vi "Error Description.vi"(8 "error in (no error)":errorcluster, 10 "Code":i32) -> (0 "error out":errorcluster, 2 "Description":string)   [LabVIEW 8.6, in "ZTScopeM.lvlib"]
doc: "Query an error code's string description\n\nNote: These are instrument error codes not VISA error codes."
uses:
  ZTScopeM.lvlib
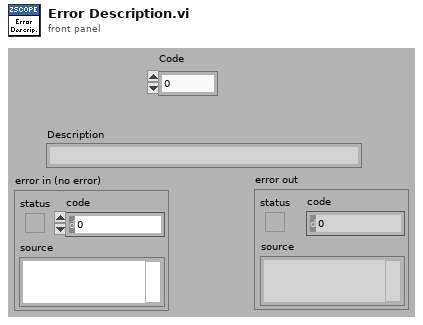
[diagram p1: front panel]
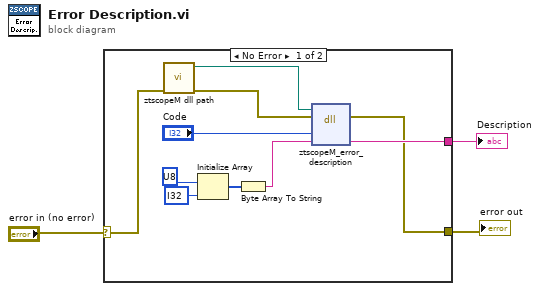
[diagram p0: block diagram]
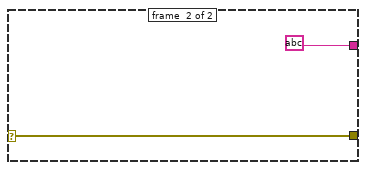
[diagram p2: hidden frame]
diagram:
  n1 = case shown="No Error" "error in (no error)" {
    selector: "error in (no error)" -> [w6 w15]
    tunnel: [w12 string ?] -> w3
    tunnel: [w4 w15] -> w1
    frame #0 {
      n2 = call "ztscopeM dll path.vi"("error in (no error)"=w6) -> ("error out"=w5:errorcluster, "<instrument>.dll path"=w7:path)  [unwired: 9 in]
      n3 = Initialize Array(u8 ?, i32 ? ("dimension size")) -> (w10:u8[])
      n4 = Byte Array To String(unsigned byte array=w10) -> (string=w9:string)
      n5 = dll-call lib="C:/Program Files (x86)/National Instruments/LabVIEW 2013/instr.lib/ztscopem/ztscopeM.dll" fn="ztscopeM_error_description"(path in=w7, error in=w5, "code"="Code", "description"=w9) -> (error out=w4:errorcluster, "description"=w12:string)  [unwired: 3 in, 1 out]
    }
    frame #1 {
    }
  }
  "Description" <- w3
  "error out" <- w1
